vi "UDSGetGenealogy.vi"(8 "error in (no error)":errorcluster, 10 "GenealogyItemsToRead":T2[](array[typedef]), 11 "SessionID":string) -> (0 "error Out":errorcluster, 2 "Success?":bool, 3 "ReadGenealogyData":T1[](array[typedef]))   [LabVIEW 2021, in "Lunar UDS CAN.lvlib"]
uses:
  Lunar UDS CAN.lvlib
  Controls/UDSGenealogyItems.ctl
  Controls/UDSReadData.ctl
  Controls/UDSActions.ctl
  b0d7efcd-a93b-4fdf-a665-c907a561f6a4.vi
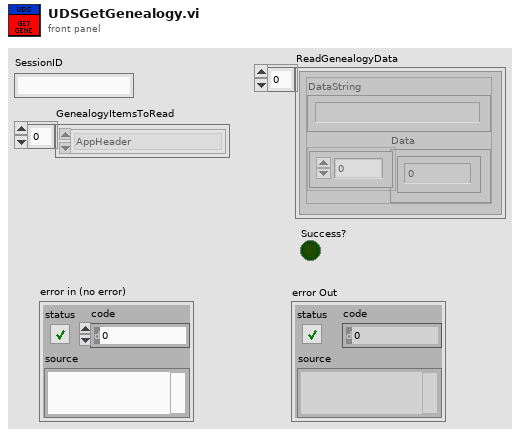
[diagram p1: front panel]
types:
  T1 = typedef "Lunar UDS CAN.lvlib/UDSReadData.ctl" = cluster{"DataString":string, "Data":i32[]}
  T2 = typedef "Lunar UDS CAN.lvlib/UDSGenealogyItems.ctl" = enum16{"AppHeader", "Genealogy Block Init", "Genealogy Block", "Board Part Number", "Board Serial Number", "Aux1 Part Number", "Aux1 Serial Number", "Aux2 Part Number", "Aux2 Serial Number", "Config Block Init", "Config Block", "Calibration Block Init", "Calibration Block", "Node Data Block Init", "Node Data Block", "Can Bus Instance"}
  T3 = typedef "Lunar UDS CAN.lvlib/UDSActions.ctl" = enum16{"Open Session", "Connect To Diagnostic Session", "Send Tester Present", "ECU Reset", "Write String Data", "Write Byte Data", "Read Data", "Close Session", "Close All Sessions"}
  T4 = typedef "Lunar UDS CAN.lvlib/UDSGenealoogyItemData.ctl" = cluster{"ID":i32, "ReadOnly":bool, "WriteOnly":bool, "Register Size":i32}
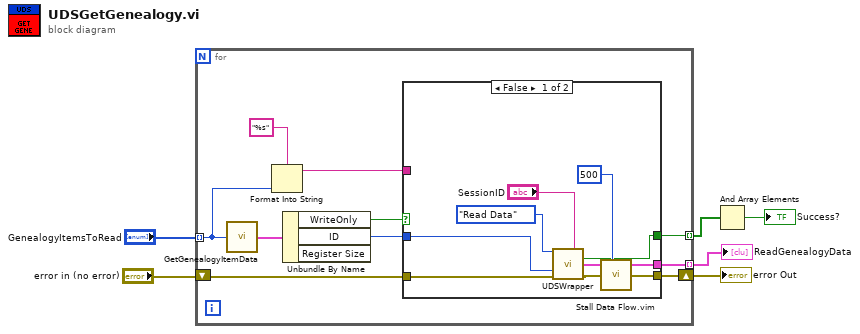
[diagram p0: block diagram]
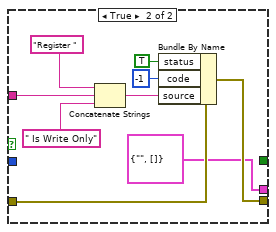
[diagram p2: hidden frame]
diagram:
  n1 = for {
    tunnel: "GenealogyItemsToRead" -> [w11] mode=indexing
    shift-right: [w12] -> w4
    shift-left: "error in (no error)" -> [w13]
    tunnel: [w8] -> w3 mode=indexing
    tunnel: [w7] -> w2 mode=indexing
    n2 = call "GetGenealogyItemData.vi"("Genealogy Item"=w11) -> ("GenealogyItemData"=w16:T4)
    n3 = Format Into String(format string="%s" ("string (\"\")"), w11) -> (resulting string=w9:string)  [unwired: 2 in, 1 out]
    n4 = Unbundle By Name(w16) -> ("WriteOnly"=w15:bool, "ID"=w14:i32)  [unwired: 1 out]
    n5 = case shown="False" w15 {
      tunnel: w14 -> [w23 _]
      tunnel: w13 -> [w24 w33]
      tunnel: [w20 w34] -> w12
      tunnel: w9 -> [_ w28]
      tunnel: [w21 cluster{"DataString":string, "Data":i32[]} {"DataString"="", "Data"=[]} ("Read Data")] -> w8
      tunnel: [w18 _] -> w7
      frame False {
        n6 = call "UDSWrapper.vi"("UDS Action"=UDSActions."Read Data", "SessionID"="SessionID", "ID"=w23, "error in (no error)"=w24) -> ("Success ?"=w18:bool, "Read Data"=w21:T1, "error out"=w22:errorcluster)  [unwired: 9 in]
        n7 = call "Stall Data Flow.vim"("value in"=w22, "milliseconds to wait"=u32 500) -> ("value out"=w20:errorcluster)  [unwired: 1 out]
      }
      frame True {
        n8 = Concatenate Strings("Register " ("string"), w28, " Is Write Only" ("string")) -> (w30:string)
        n9 = Bundle By Name(cluster=w33, "status"=TRUE, "code"=-1, "source"=w30) -> (w34:errorcluster)
      }
    }
  }
  "error Out" <- w4
  "ReadGenealogyData" <- w3
  n10 = And Array Elements(Boolean array=w2) -> (logical AND=→"Success?":bool)
